vi "Stringhandling(SubVI)0.0.2.vi"(0 "Slide (Eingang)":refnum<vi>, 1 "Numerisch (Eingang)":i32, 3 "VISA-Referenz (Eingang)":refnum<visa-resource-name>, 4 "MessFrequenz [Hz]":dbl, 5 "Bytes at Port":u32, 7 "Fehler (Eingang, kein Fehler)":errorcluster, 8 "Cyclecounter (Eingang)":i32, 9 "Rolle[Hz]":dbl, 10 "Temp[°C] (Eingang)":dbl, 11 "AFR (Eingang)":dbl, 12 "String (Eingang)":string, 13 "Zündung [Hz] (Eingang)":dbl, 15 "AFR+EGT":bool) -> (14 "Lesepuffer":string="\n", 16 "Numerisch (Ausgang)":i32, 17 "String (Ausgang)":string, 18 "Temp[°C] (Ausgang)":dbl, 19 "AFR (Ausgang)":dbl, 20 "VISA-Referenz (Ausgang)":refnum<visa-resource-name>, 21 "Zündung [Hz] (Ausgang)":dbl, 23 "Rolle [Hz]":dbl, 24 "Messfrequenz [Hz]":dbl, 25 "Cyclecounter (Ausgang)":i32, 27 "Fehler (Ausgang)":errorcluster)   [LabVIEW 2014]
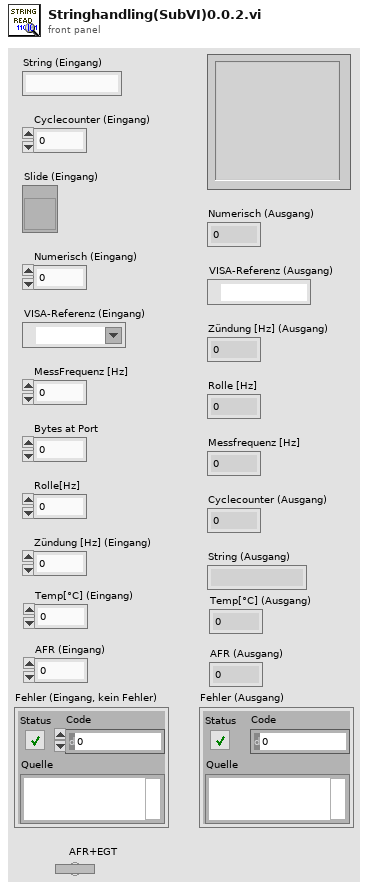
[diagram p1: front panel]
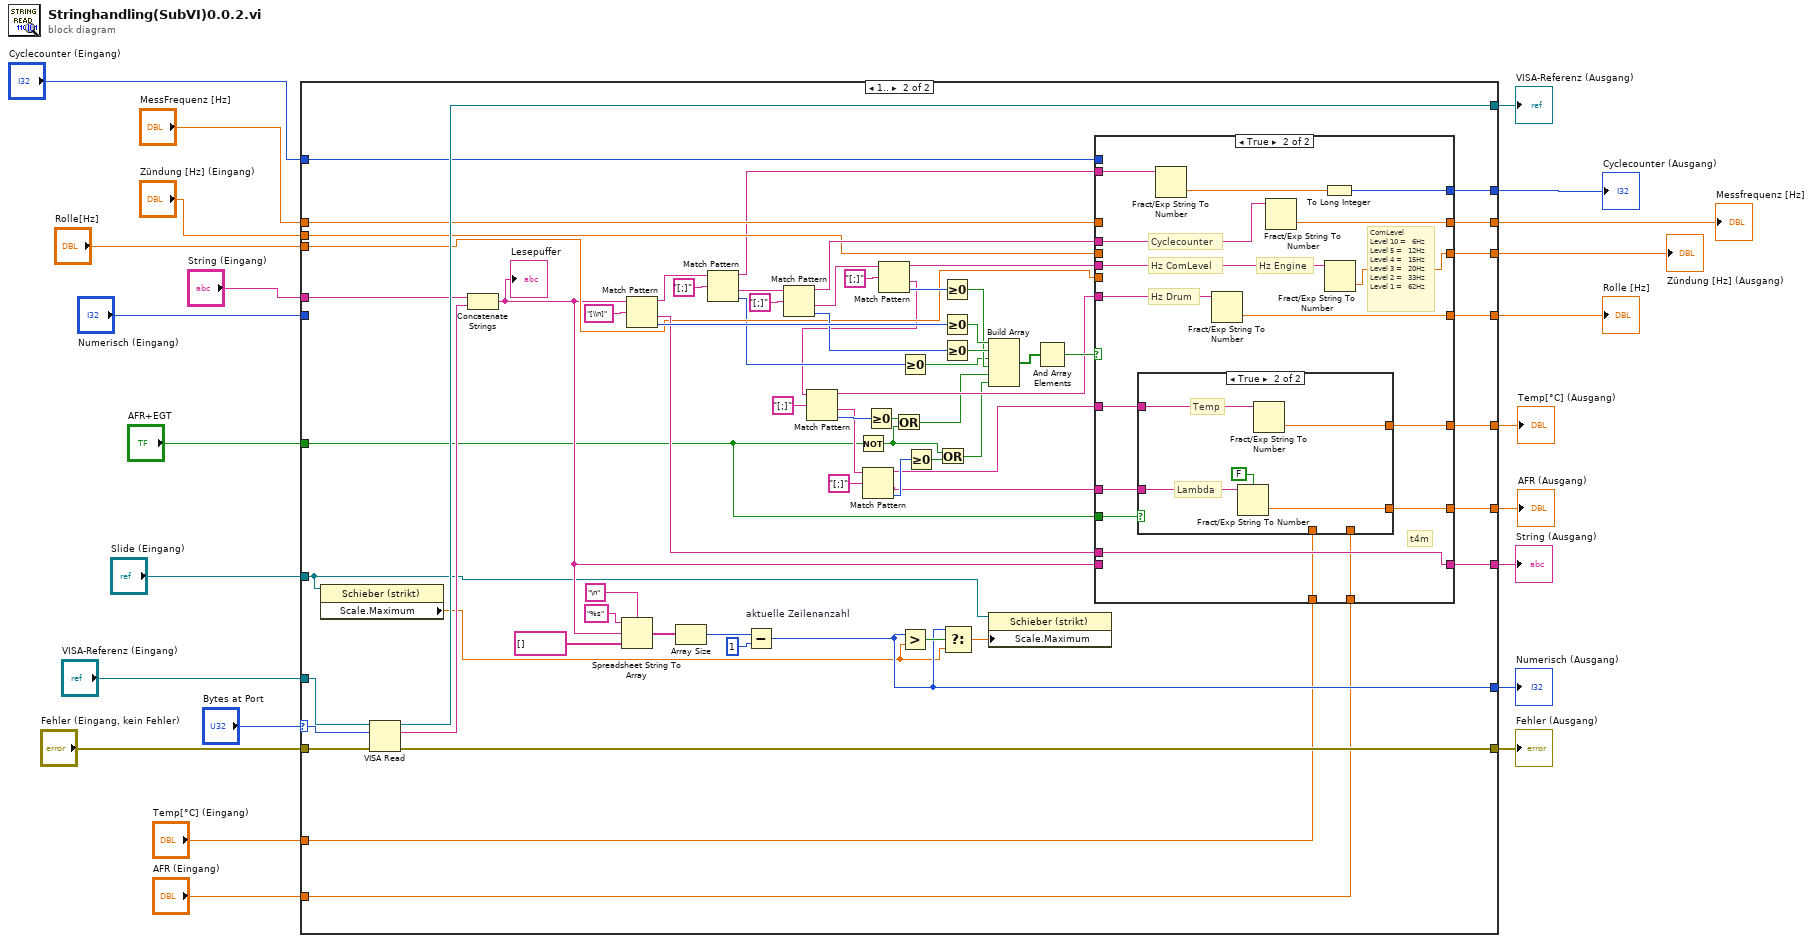
[diagram p0: block diagram]
diagram:
  n1 = case shown="1.." "Bytes at Port" {
    selector: "Bytes at Port" -> [_ w96]
    tunnel: [w27 w91] -> w15
    tunnel: [w26 w92] -> w20
    tunnel: [w31 w93] -> w13
    tunnel: [w32 w90] -> w12
    tunnel: "String (Eingang)" -> [w33 w88]
    tunnel: [w33 w86] -> w7
    tunnel: "Zündung [Hz] (Eingang)" -> [w32 w78]
    tunnel: "Rolle[Hz]" -> [w31 w77]
    tunnel: [w28 w76] -> w16
    tunnel: "MessFrequenz [Hz]" -> [w28 w75]
    tunnel: "Numerisch (Eingang)" -> [w30 _]
    tunnel: [w30 w58] -> w14
    tunnel: [w29 w64] -> w17
    tunnel: "Cyclecounter (Eingang)" -> [w29 w63]
    tunnel: "VISA-Referenz (Eingang)" -> [w26 w55]
    tunnel: "Fehler (Eingang, kein Fehler)" -> [w27 w54]
    tunnel: "Slide (Eingang)" -> [_ w35]
    tunnel: [w25 w44] -> w5
    tunnel: [w24 w43] -> w4
    tunnel: "Temp[°C] (Eingang)" -> [w25 w42]
    tunnel: "AFR (Eingang)" -> [w24 w41]
    tunnel: "AFR+EGT" -> [_ w34]
    frame 0, Default {
      # "No data in from serial port - Nothing to do."
    }
    frame 1.. {
      n2 = property on="Eigenschaftsknoten" class="Schieber (strikt)"(reference=w35) -> ("Scale.Maximum"=w57:dbl)  [unwired: 1 in, 2 out]
      n3 = VISA Read(VISA resource name=w55, byte count=w96, error in (no error)=w54) -> (VISA resource name out=w92:refnum<visa-resource-name>, read buffer=w89:string, error out=w91:errorcluster)  [unwired: 1 out]
      n4 = Concatenate Strings(w88, w89) -> (w60:string)
      "Lesepuffer" <- w60
      n5 = Spreadsheet String To Array(delimiter (Tab)="\n" ("regular expression"), format string="%s" ("regular expression"), spreadsheet string=w60, array type (2D Dbl)=string[] [] ("Array 2")) -> (array=w69:string[])
      n6 = Match Pattern(string=w60, regular expression="[\\n]") -> (before substring=w67:string, after substring=w87:string, offset past match=w100:i32)  [unwired: 1 in, 1 out]
      n7 = Array Size(array=w69) -> (size(s)=w73:i32)
      n8 = Match Pattern(string=w67, regular expression="[;]") -> (before substring=w65:string, after substring=w66:string, offset past match=w62:i32)  [unwired: 1 in, 1 out]
      n9 = Subtract "aktuelle Zeilenanzahl"(x=w73, y=1) -> (x-y=w58:i32)
      n10 = Match Pattern(string=w66, regular expression="[;]") -> (before substring=w95:string, after substring=w98:string, offset past match=w84:i32)  [unwired: 1 in, 1 out]
      n11 = Not(x=w34) -> (.not. x?=w36:bool)
      n12 = Match Pattern(string=w98, regular expression="[;]") -> (before substring=w94:string, after substring=w50:string, offset past match=w82:i32)  [unwired: 1 in, 1 out]
      n13 = Match Pattern(string=w50, regular expression="[;]") -> (before substring=w51:string, after substring=w47:string, offset past match=w52:i32)  [unwired: 1 in, 1 out]
      n14 = Match Pattern(string=w47, regular expression="[;]") -> (before substring=w45:string, after substring=w46:string, offset past match=w48:i32)  [unwired: 1 in, 1 out]
      n15 = Greater Or Equal To 0?(x=w52) -> (x >= 0?=w40:bool)
      n16 = Or(x=w40, y=w36) -> (x .or. y?=w39:bool)
      n17 = Greater Or Equal To 0?(x=w62) -> (x >= 0?=w61:bool)
      n18 = Greater?(x=w58, y=w57) -> (0:w59:bool)
      n19 = Greater Or Equal To 0?(x=w48) -> (x >= 0?=w38:bool)
      n20 = Or(x=w36, y=w38) -> (x .or. y?=w37:bool)
      n21 = Greater Or Equal To 0?(x=w82) -> (x >= 0?=w81:bool)
      n22 = Greater Or Equal To 0?(x=w100) -> (x >= 0?=w85:bool)
      n23 = Greater Or Equal To 0?(x=w84) -> (x >= 0?=w83:bool)
      n24 = Select(t=w58, s=w59, f=w57) -> (s? t:f=w56:dbl)
      n25 = Build Array(w85, w83, w61, w81, w39, w37) -> (w80:bool[])
      n26 = property on="Eigenschaftsknoten" class="Schieber (strikt)"(reference=w35, "Scale.Maximum"=w56) -> ()  [unwired: 1 in, 2 out]
      n27 = And Array Elements(Boolean array=w80) -> (logical AND=w79:bool)
      n28 = case shown="True" w79 {
        tunnel: w95 -> [_ w120]
        tunnel: w94 -> [_ w125]
        tunnel: w51 -> [_ w124]
        tunnel: [w106 w123] -> w93
        tunnel: [w107 w122] -> w90
        tunnel: w87 -> [_ w121]
        tunnel: [w108 w121] -> w86
        tunnel: w60 -> [w108 _]
        tunnel: w78 -> [w107 _]
        tunnel: w77 -> [w106 _]
        tunnel: [w105 w119] -> w76
        tunnel: w75 -> [w105 _]
        tunnel: w65 -> [_ w118]
        tunnel: [w104 w116] -> w64
        tunnel: w63 -> [w104 _]
        tunnel: w46 -> [_ w115]
        tunnel: w45 -> [_ w114]
        tunnel: [w103 w113] -> w44
        tunnel: [w102 w112] -> w43
        tunnel: w42 -> [w103 w109]
        tunnel: w41 -> [w102 w110]
        tunnel: w34 -> [_ w111]
        frame False {
        }
        frame True {
          # "Cyclecounter"
          # "Hz ComLevel"
          # "ComLevel\nLevel 10 =   6Hz \nLevel 5 =   12Hz \nLevel 4 =   15Hz\nLevel 3 =   20Hz\nLevel 2 =   33Hz\nLevel 1 =   62Hz"
          # "Hz Drum"
          # "Hz Engine"
          # "t4m"
          n29 = case shown="True" w111 {
            tunnel: w115 -> [_ w131]
            tunnel: w114 -> [_ w130]
            tunnel: [w126 w129] -> w113
            tunnel: [w127 w128] -> w112
            tunnel: w110 -> [w127 _]
            tunnel: w109 -> [w126 _]
            frame False {
            }
            frame True {
              # "Temp"
              # "Lambda"
              n30 = Fract/Exp String To Number(use system decimal point (T)=FALSE, string=w131) -> (number=w128:dbl)  [unwired: 2 in, 1 out]
              n31 = Fract/Exp String To Number(string=w130) -> (number=w129:dbl)  [unwired: 3 in, 1 out]
            }
          }
          n32 = Fract/Exp String To Number(string=w118) -> (number=w117:dbl)  [unwired: 3 in, 1 out]
          n33 = Fract/Exp String To Number(string=w124) -> (number=w123:dbl)  [unwired: 3 in, 1 out]
          n34 = Fract/Exp String To Number(string=w120) -> (number=w119:dbl)  [unwired: 3 in, 1 out]
          n35 = To Long Integer(number=w117) -> (32bit integer=w116:i32)
          n36 = Fract/Exp String To Number(string=w125) -> (number=w122:dbl)  [unwired: 3 in, 1 out]
        }
      }
    }
  }
  "VISA-Referenz (Ausgang)" <- w20
  "Cyclecounter (Ausgang)" <- w17
  "Messfrequenz [Hz]" <- w16
  "Fehler (Ausgang)" <- w15
  "Numerisch (Ausgang)" <- w14
  "Rolle [Hz]" <- w13
  "Zündung [Hz] (Ausgang)" <- w12
  "String (Ausgang)" <- w7
  "AFR (Ausgang)" <- w4
  "Temp[°C] (Ausgang)" <- w5
